vi "鼠标坐标记录.vi"() -> ()   [LabVIEW 2018]
panel:
  out "坐标":cluster{"垂直":dbl, "水平2":dbl}
  in  "停止":bool
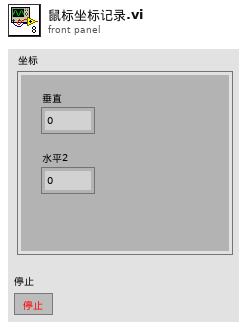
[diagram p1: front panel]
types:
  T1 = typedef "LVPoint32TypeDef.ctl" = cluster{"Horizontal":i32, "Vertical":i32}
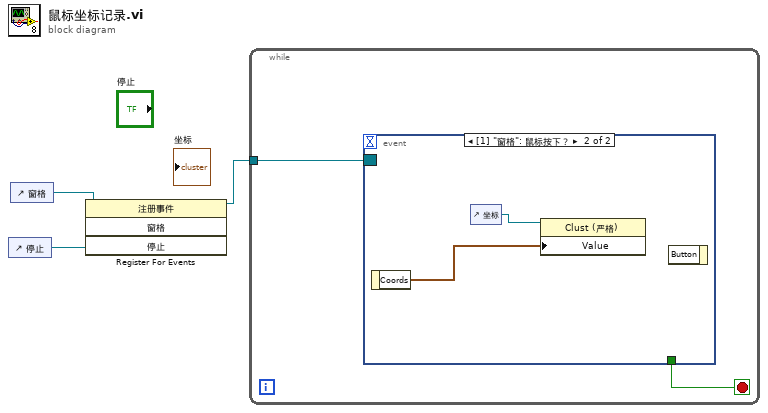
[diagram p0: block diagram]
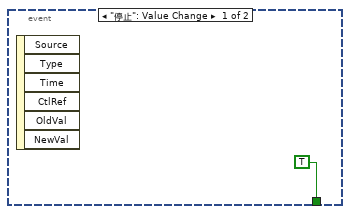
[diagram p2: hidden frame]
diagram:
  n1 = control-ref of="停止"() -> (w2:refnum<vi>)
  n2 = control-ref of="窗格"() -> (w3:refnum<vi>)
  n3 = register-events(w3, w2) -> (reference out=w1:refnum<event-registration>)  [unwired: 2 in, 1 out]
  n4 = while {
    tunnel: w1 -> [w4]
    stop <- w5 stop-if-true
    n5 = event shown="[1] \"窗格\": 鼠标按下？" {
      selector: w4 -> [_ _]
      dyn-events: _ -> [_ _]
      timeout: _ -> [_ _]
      tunnel: [TRUE _] -> w5
      event "停止": Value Change {
        n6 = event-data() -> ()  [unwired: 1 in, 6 out]
      }
      event Mouse Down? {
        n7 = event-data() -> ("Coords"=w7:T1)  [unwired: 1 in]
        n8 = control-ref of="坐标"() -> (w8:refnum<vi>)
        n9 = property class="Clust (严格)"(reference=w8, "Value"=w7) -> ()  [unwired: 1 in, 2 out]
        n10 = event-data() -> ()  [unwired: 2 in, 1 out]
      }
    }
  }
